vi "CRYASIOGetDriverNames.vi"(10 "Driver Count":i32, 11 "error in (no error)":errorcluster) -> (2 "Driver Name Array":string[](array[string]), 3 "error out":errorcluster)   [LabVIEW 2013]
uses:
  CRY_ASIO.dll
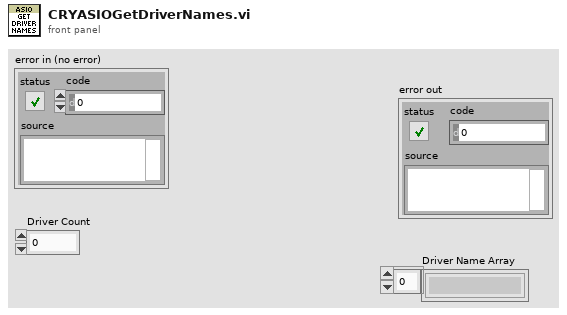
[diagram p1: front panel]
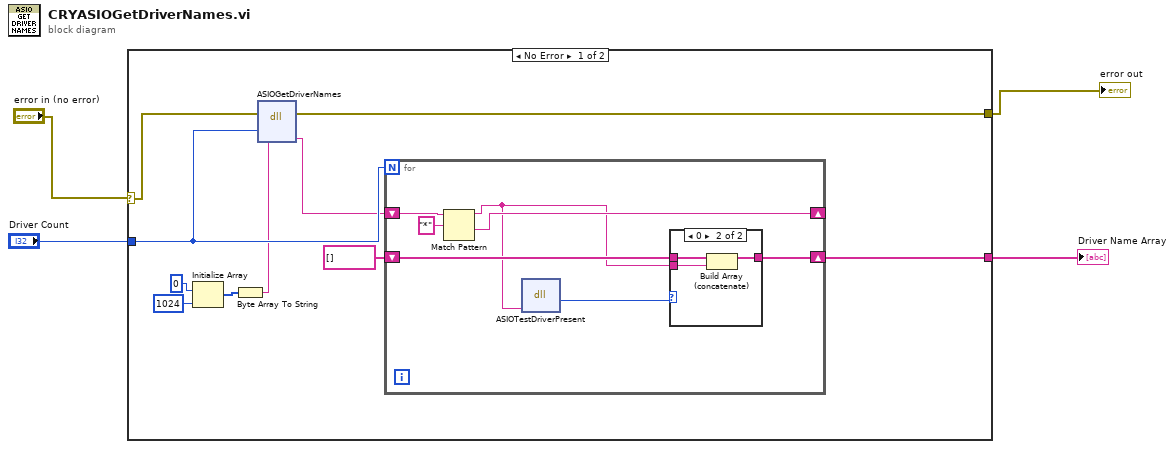
[diagram p0: block diagram]
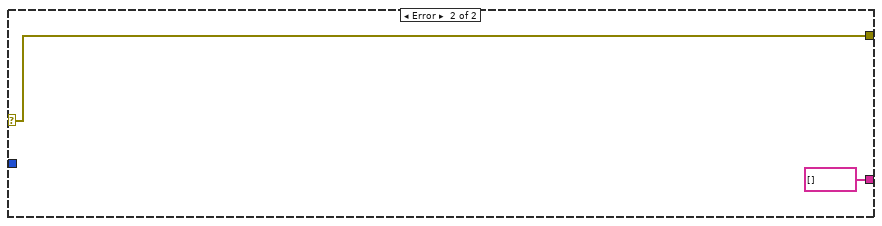
[diagram p3: hidden frame]
diagram:
  n1 = case shown="No Error" "error in (no error)" {
    selector: "error in (no error)" -> [w13 w27]
    tunnel: [w14 w27] -> w4
    tunnel: "Driver Count" -> [w12 _]
    tunnel: [w9 string[] []] -> w1
    frame No Error {
      n2 = Initialize Array(u8 0 ("dimension size"), 1024 ("dimension size")) -> (w6:u8[])
      n3 = Byte Array To String(unsigned byte array=w6) -> (string=w5:string)
      n4 = dll-call lib="D:/LabView_Project/CRY6181/CRY_ASIO.dll" fn="ASIOGetDriverNames"(error in=w13, "arg1"=w12, "arg2"=w5) -> (error out=w14:errorcluster, "arg2"=w11:string)  [unwired: 4 in, 1 out]
      n5 = for {
        N: w12 -> [_]
        shift-right: [w19] -> _
        shift-left: w11 -> [w20]
        shift-right: [w18] -> w9
        shift-left: string[] [] -> [w17]
        n6 = Match Pattern(string=w20, regular expression="*") -> (before substring=w16:string, after substring=w19:string)  [unwired: 1 in, 2 out]
        n7 = dll-call lib="D:/LabView_Project/CRY6181/CRY_ASIO.dll" fn="ASIOTestDriverPresent"("arg1"=w16) -> ("return type"=w15:i32)  [unwired: 4 in, 2 out]
        n8 = case shown="0" w15 {
          tunnel: [w22 w25] -> w18
          tunnel: w16 -> [_ w24]
          tunnel: w17 -> [w22 w23]
          frame 1, Default {
          }
          frame 0 {
            n9 = Build Array (concatenate)(w23, w24) -> (w25:string[])
          }
        }
      }
    }
    frame Error {
    }
  }
  "error out" <- w4
  "Driver Name Array" <- w1
